vi "Initialize.vi"(8 "error in (no error)":errorcluster, 11 "State in":T1={"State"=enum."Idle", "Start Time"=timestamp(0 s since 1904-01-01), "Configuration"={"Cycle Period"=0.0, "Ismatech"={"VISA resource name"="", "Simulated?"=FALSE, "Pump Number"=1.0, "Reverse?"=FALSE}, "Masterflex"={"VISA resource name"="", "Simulated?"=FALSE, "Pump Number"=1.0, "Reverse?"=FALSE}, "Mettler"={"VISA resource name"="", "Simulated?"=FALSE}, "Bronkhorst M13 Flow Meter"={"VISA resource name"="", "Simulated?"=FALSE}, "PID 2 Parameters"={"Input Device"=enum."Bronkhorst M13", "Output Device"=enum."Ismatec ISM 831C", "Setpoint"=0.0, "PID gains"={"proportional gain (Kc)"=1.0, "integral time (Ti, min)"=0.01, "derivative time (Td, min)"=0.0}}, "Manual Entry"=0.0, "Auto?"=TRUE, "output range"={"output high"=100.0, "output low"=0.0}, "Bronkhorst M14"={"VISA resource name"="", "Simulated?"=FALSE}, "Tacmina Settings"={"Analog DAQ Task"="", "Digital DAQ Task"=""}, "KNF SIMDOS Settings"={"VISA resource name"="", "Simulated?"=TRUE}, "ASIA Pump C"={"ASIA Pump #"=0, "channel"=0, "Simulated"=FALSE}, "VICI Settings"={"VISA resource name"="", "Simulated?"=FALSE, "Pump Letter"="", "Reverse?"=FALSE}, "FLOM Settings"={"VISA resource name"="", "Simulated?"=TRUE, "Pump Number"=0.0}, "SSI PR Settings"={"VISA resource name"="", "Simulated?"=FALSE}}, "Current Time"=timestamp(0 s since 1904-01-01), "PID 1 Parameters"={"Setpoint"=0.0, "PID gains"={"proportional gain (Kc)"=1.0, "integral time (Ti, min)"=0.01, "derivative time (Td, min)"=0.0}}, "First Iteration"=FALSE, "Data"={"Flowmeter Output"=0.0, "Density"=0.0, "FL Temp"=0.0, "Scale Output (g)"=0.0, "Scale Rate of Change (g/min)"=0.0, "PID 1 Output"=0.0, "PID 2 Process Variable"=0.0, "PID 2 output"=0.0, "Pump Flow"=0.0, "Pump Pressure"=0.0}, "Process Name"="", "Pump On?"=enum."Off", "Input Error"=FALSE, "Output Error"=FALSE, "Log Started"=FALSE, "Current Setpoint"=0.0} {"PID 1 Parameters"."PID gains"."derivative time (Td, min)" format="%.3f"; "PID 1 Parameters"."PID gains"."integral time (Ti, min)" format="%.3f"; "PID 1 Parameters"."PID gains"."proportional gain (Kc)" format="%.3f"; "Configuration"."output range"."output low" min=0.0 max=100.0 format="%.2f"; "Configuration"."output range"."output high" format="%.2f"; "Configuration"."PID 2 Parameters"."PID gains"."derivative time (Td, min)" format="%.3f"; "Configuration"."PID 2 Parameters"."PID gains"."integral time (Ti, min)" format="%.3f"; "Configuration"."PID 2 Parameters"."PID gains"."proportional gain (Kc)" format="%.3f"; "Configuration"."ASIA Pump C"."channel" min=0 max=1 step=1; "Configuration"."Ismatech"."Pump Number" min=1.0 max=20.0 step=1.0; "Configuration"."Masterflex"."Pump Number" min=1.0 max=20.0 step=1.0}) -> (0 "error out":errorcluster, 1 "Pump Initialized":bool, 3 "State out":T1={"State"=enum."Idle", "Start Time"=timestamp(0 s since 1904-01-01), "Configuration"={"Cycle Period"=0.0, "Ismatech"={"VISA resource name"="", "Simulated?"=FALSE, "Pump Number"=1.0, "Reverse?"=FALSE}, "Masterflex"={"VISA resource name"="", "Simulated?"=FALSE, "Pump Number"=1.0, "Reverse?"=FALSE}, "Mettler"={"VISA resource name"="", "Simulated?"=FALSE}, "Bronkhorst M13 Flow Meter"={"VISA resource name"="", "Simulated?"=FALSE}, "PID 2 Parameters"={"Input Device"=enum."Bronkhorst M13", "Output Device"=enum."Ismatec ISM 831C", "Setpoint"=0.0, "PID gains"={"proportional gain (Kc)"=1.0, "integral time (Ti, min)"=0.01, "derivative time (Td, min)"=0.0}}, "Manual Entry"=0.0, "Auto?"=TRUE, "output range"={"output high"=100.0, "output low"=0.0}, "Bronkhorst M14"={"VISA resource name"="", "Simulated?"=FALSE}, "Tacmina Settings"={"Analog DAQ Task"="", "Digital DAQ Task"=""}, "KNF SIMDOS Settings"={"VISA resource name"="", "Simulated?"=TRUE}, "ASIA Pump C"={"ASIA Pump #"=0, "channel"=0, "Simulated"=FALSE}, "VICI Settings"={"VISA resource name"="", "Simulated?"=FALSE, "Pump Letter"="", "Reverse?"=FALSE}, "FLOM Settings"={"VISA resource name"="", "Simulated?"=TRUE, "Pump Number"=0.0}, "SSI PR Settings"={"VISA resource name"="", "Simulated?"=FALSE}}, "Current Time"=timestamp(0 s since 1904-01-01), "PID 1 Parameters"={"Setpoint"=0.0, "PID gains"={"proportional gain (Kc)"=1.0, "integral time (Ti, min)"=0.01, "derivative time (Td, min)"=0.0}}, "First Iteration"=FALSE, "Data"={"Flowmeter Output"=0.0, "Density"=0.0, "FL Temp"=0.0, "Scale Output (g)"=0.0, "Scale Rate of Change (g/min)"=0.0, "PID 1 Output"=0.0, "PID 2 Process Variable"=0.0, "PID 2 output"=0.0, "Pump Flow"=0.0, "Pump Pressure"=0.0}, "Process Name"="", "Pump On?"=enum."Off", "Input Error"=FALSE, "Output Error"=FALSE, "Log Started"=FALSE, "Current Setpoint"=0.0} {"PID 1 Parameters"."PID gains"."derivative time (Td, min)" format="%.3f"; "PID 1 Parameters"."PID gains"."integral time (Ti, min)" format="%.3f"; "PID 1 Parameters"."PID gains"."proportional gain (Kc)" format="%.3f"; "Configuration"."output range"."output low" min=0.0 max=100.0 format="%.2f"; "Configuration"."output range"."output high" format="%.2f"; "Configuration"."PID 2 Parameters"."PID gains"."derivative time (Td, min)" format="%.3f"; "Configuration"."PID 2 Parameters"."PID gains"."integral time (Ti, min)" format="%.3f"; "Configuration"."PID 2 Parameters"."PID gains"."proportional gain (Kc)" format="%.3f"; "Configuration"."ASIA Pump C"."channel" min=0 max=1 step=1; "Configuration"."Ismatech"."Pump Number" min=1.0 max=20.0 step=1.0; "Configuration"."Masterflex"."Pump Number" min=1.0 max=20.0 step=1.0})   [LabVIEW 2018, in "Feed Module.lvlib" / "Feed Module Engine.lvlib"]
uses:
  Feed Module Engine.lvlib
  State Cluster.ctl
  State Enum.ctl
  Feed Module/Controls/Feed Module Settings Cluster.ctl
  Ismatec ISM 831C/Controls/Ismatech Settings Cluster.ctl
  Masterflex 7550-30/Controls/Settings Cluster.ctl
  Mettler Toledo/Controls/Settings Cluster.ctl
  Bronkhorst M13 Flow Meter/Settings Cluster.ctl
  PID 2 Parameters Cluster.ctl
  PID Input Enum.ctl
  PID 2 Output Enum.ctl
  Tacmina QI/Tacmina QI DAQ Setting.ctl
  KNF Pump/Settings Cluster plus SIMDOS.ctl
  ASIA Pump/Pump Settings.ctl
  VICI M50 Party Mode/Settings Cluster.ctl
  FLOM Pump/Settings Cluster.ctl
  SSI PR Class/SSI PR Settings Cluster.ctl
  PID 1 Parameters Cluster.ctl
  Pump Module Folder/Measure Instrument/Pump Settings Cluster.ctl
  Tag VIs/Tag FGV Operation Enum.ctl
  Mettler Toledo/Mettler Toledo.lvlib
  Bronkhorst M13 Flow Meter/Bronkhorst M13 Flow Meter.lvlib
  Shared Variables/Dynamic Shared Variables.lvlib
  Bronkhorst M14 Flow Meter/Bronkhorst M14 Flow Meter.lvlib
  Pump Module Folder/Measure Instrument/Pump Module Engine.lvlib
  SSI PR Class/SSI PR Pump.lvlib
  FLOM Pump/FLOM Pump.lvlib
  ASIA Pump.lvlib
  KNF Pump/KNF SIMDOS.lvlib
  Tacmina QI/Tacmina QI.lvlib
  VICI M50 Party Mode/VICI M6 M50 Party Mode.lvlib
  Ismatec ISM 831C/Ismatec ISM 831C.lvlib
  Masterflex 7550-30/Masterflex 7550-30.lvlib
  Pump Module Folder/Pump Module.lvlib
  Feed Module/Feed Module.lvlib
panel:
  out "Input Initialized":bool
  # "Output Instruments"
  # "Input Instruments"
  # "Output Instruments"
  # "Input Instruments"
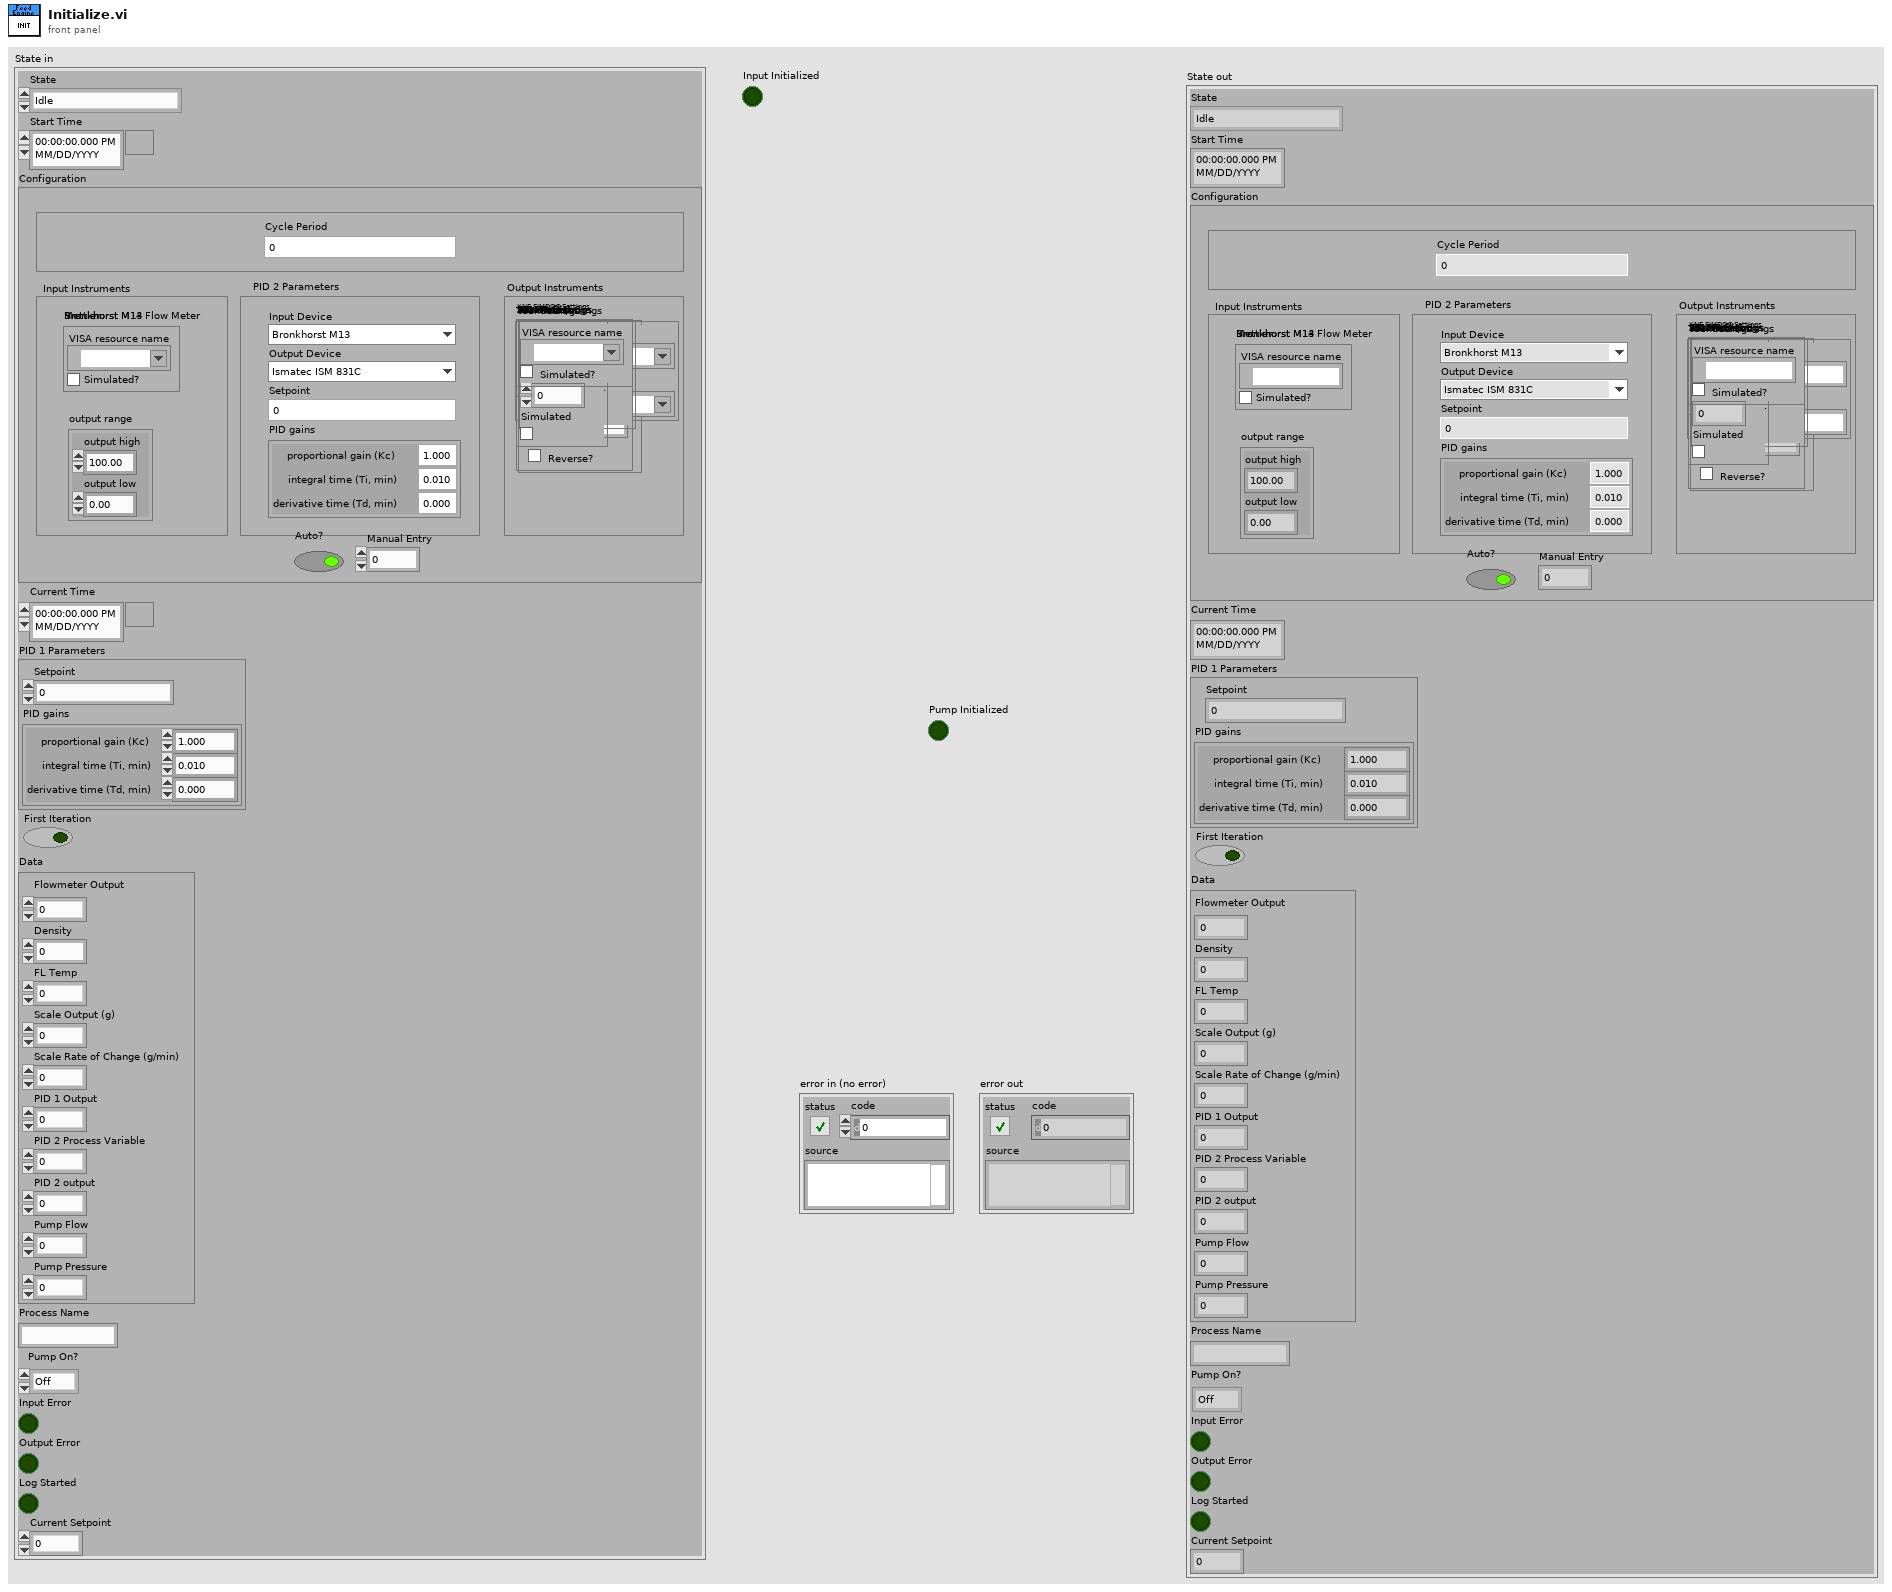
[diagram p1: front panel]
types:
  T1 = typedef "Feed Module.lvlib/Feed Module Engine.lvlib/State Cluster.ctl" = cluster{"State":T2, "Start Time":timestamp, "Configuration":T3, "Current Time":timestamp, "PID 1 Parameters":T17, "First Iteration":bool, "Data":cluster{"Flowmeter Output":dbl, "Density":dbl, "FL Temp":dbl, "Scale Output (g)":dbl, "Scale Rate of Change (g/min)":dbl, "PID 1 Output":dbl, "PID 2 Process Variable":dbl, "PID 2 output":dbl, "Pump Flow":dbl, "Pump Pressure":dbl}, "Process Name":string, "Pump On?":enum16{"Off", "On", "Not Initialized"}, "Input Error":bool, "Output Error":bool, "Log Started":bool, "Current Setpoint":dbl}
  T2 = typedef "Feed Module.lvlib/Feed Module Engine.lvlib/State Enum.ctl" = enum16{"Measuring", "Idle", "Paused"}
  T3 = typedef "Feed Module.lvlib/Feed Module Settings Cluster.ctl" = cluster{"Cycle Period":dbl, "Ismatech":T4, "Masterflex":T5, "Mettler":T6, "Bronkhorst M13 Flow Meter":T7, "PID 2 Parameters":T8, "Manual Entry":dbl, "Auto?":bool, "output range":cluster{"output high":dbl, "output low":dbl}, "Bronkhorst M14":T6, "Tacmina Settings":T11, "KNF SIMDOS Settings":T12, "ASIA Pump C":T13, "VICI Settings":T14, "FLOM Settings":T15, "SSI PR Settings":T16}
  T4 = typedef "Ismatec ISM 831C.lvlib/Ismatech Settings Cluster.ctl" = cluster{"VISA resource name":refnum<visa-resource-name>, "Simulated?":bool, "Pump Number":dbl, "Reverse?":bool}
  T5 = typedef "Masterflex 7550-30.lvlib/Settings Cluster.ctl" = cluster{"VISA resource name":refnum<visa-resource-name>, "Simulated?":bool, "Pump Number":dbl, "Reverse?":bool}
  T6 = typedef "Mettler Toledo.lvlib/Settings Cluster.ctl" = cluster{"VISA resource name":refnum<visa-resource-name>, "Simulated?":bool}
  T7 = typedef "Bronkhorst M13 Flow Meter.lvlib/Settings Cluster.ctl" = cluster{"VISA resource name":refnum<visa-resource-name>, "Simulated?":bool}
  T8 = typedef "PID 2 Parameters Cluster.ctl" = cluster{"Input Device":T9, "Output Device":T10, "Setpoint":dbl, "PID gains":cluster{"proportional gain (Kc)":dbl, "integral time (Ti, min)":dbl, "derivative time (Td, min)":dbl}}
  T9 = typedef "PID Input Enum.ctl" = enum16{"Default", "Bronkhorst M13", "Bronkhorst M14", "Scale Rate of Change"}
  T10 = typedef "PID 2 Output Enum.ctl" = enum16{"Default", "Ismatec ISM 831C", "Masterflex 7550-30", "VICI", "Tacmina QI", "KNF SIMDOS", "ASIA Type C", "FLOM UI-22-11", "SSI PR"}
  T11 = typedef "Tacmina QI.lvlib/Tacmina QI DAQ Setting.ctl" = cluster{"Analog DAQ Task":refnum<k21>, "Digital DAQ Task":refnum<k21>}
  T12 = typedef "KNF SIMDOS.lvlib/Settings Cluster plus SIMDOS.ctl" = cluster{"VISA resource name":refnum<visa-resource-name>, "Simulated?":bool}
  T13 = typedef "ASIA Pump.lvlib/Pump Settings.ctl" = cluster{"ASIA Pump #":i32, "channel":i32, "Simulated":bool}
  T14 = typedef "VICI M6 M50 Party Mode.lvlib/Settings Cluster.ctl" = cluster{"VISA resource name":refnum<visa-resource-name>, "Simulated?":bool, "Pump Letter":string, "Reverse?":bool}
  T15 = typedef "FLOM Pump.lvlib/Settings Cluster.ctl" = cluster{"VISA resource name":refnum<visa-resource-name>, "Simulated?":bool, "Pump Number":dbl}
  T16 = typedef "SSI PR Pump.lvlib/SSI PR Settings Cluster.ctl" = cluster{"VISA resource name":refnum<visa-resource-name>, "Simulated?":bool}
  T17 = typedef "PID 1 Parameters Cluster.ctl" = cluster{"Setpoint":dbl, "PID gains":cluster{"proportional gain (Kc)":dbl, "integral time (Ti, min)":dbl, "derivative time (Td, min)":dbl}}
  T18 = typedef "Pump Module.lvlib/Pump Settings Cluster.ctl" = cluster{"Output Device":T10, "Masterflex":T5, "Ismatech":T4, "VICI Settings":T14, "Tacmina Settings":T11, "KNF SIMDOS Settings":T12, "ASIA Pump C":T13, "FLOM Settings":T15, "SSI PR Settings":T16}
  T19 = typedef "Tag FGV Operation Enum.ctl" = enum16{"Init", "Set Notification Queue", "Create Tag", "Commit", "Write Tag (Numeric)", "Write Tag (Boolean)", "Read All Tags", "Read One Tag", "Delete Tag Category", "Set Alarm Parameters (Numeric)", "Set Alarm Parameters (Boolean)", "Enable All Alarms", "Disable All Alarms", "Delete All Tags", "Read Alarms", "Ack Alarm", "Read Alarm Parameters (Numeric)", "Read Alarm Parameters (Boolean)"}
  T20 = typedef "Feed Module.lvlib/Feed Module Tag Names Cluster.ctl" = cluster{"Pump Flow Tag":string, "PID 2 Out Tag":string, "Scale Tag":string, "Density Tag":string, "FL Temp":string, "Input Device Tag":string, "Output Device Tag":string, "Pump's Flow":string, "Pump's Pressure":string, "Overpressure Tag":string}
  T21 = typedef "Bronkhorst M14 Flow Meter.lvlib/Settings Cluster.ctl" = cluster{"VISA resource name":refnum<visa-resource-name>, "Simulated?":bool}
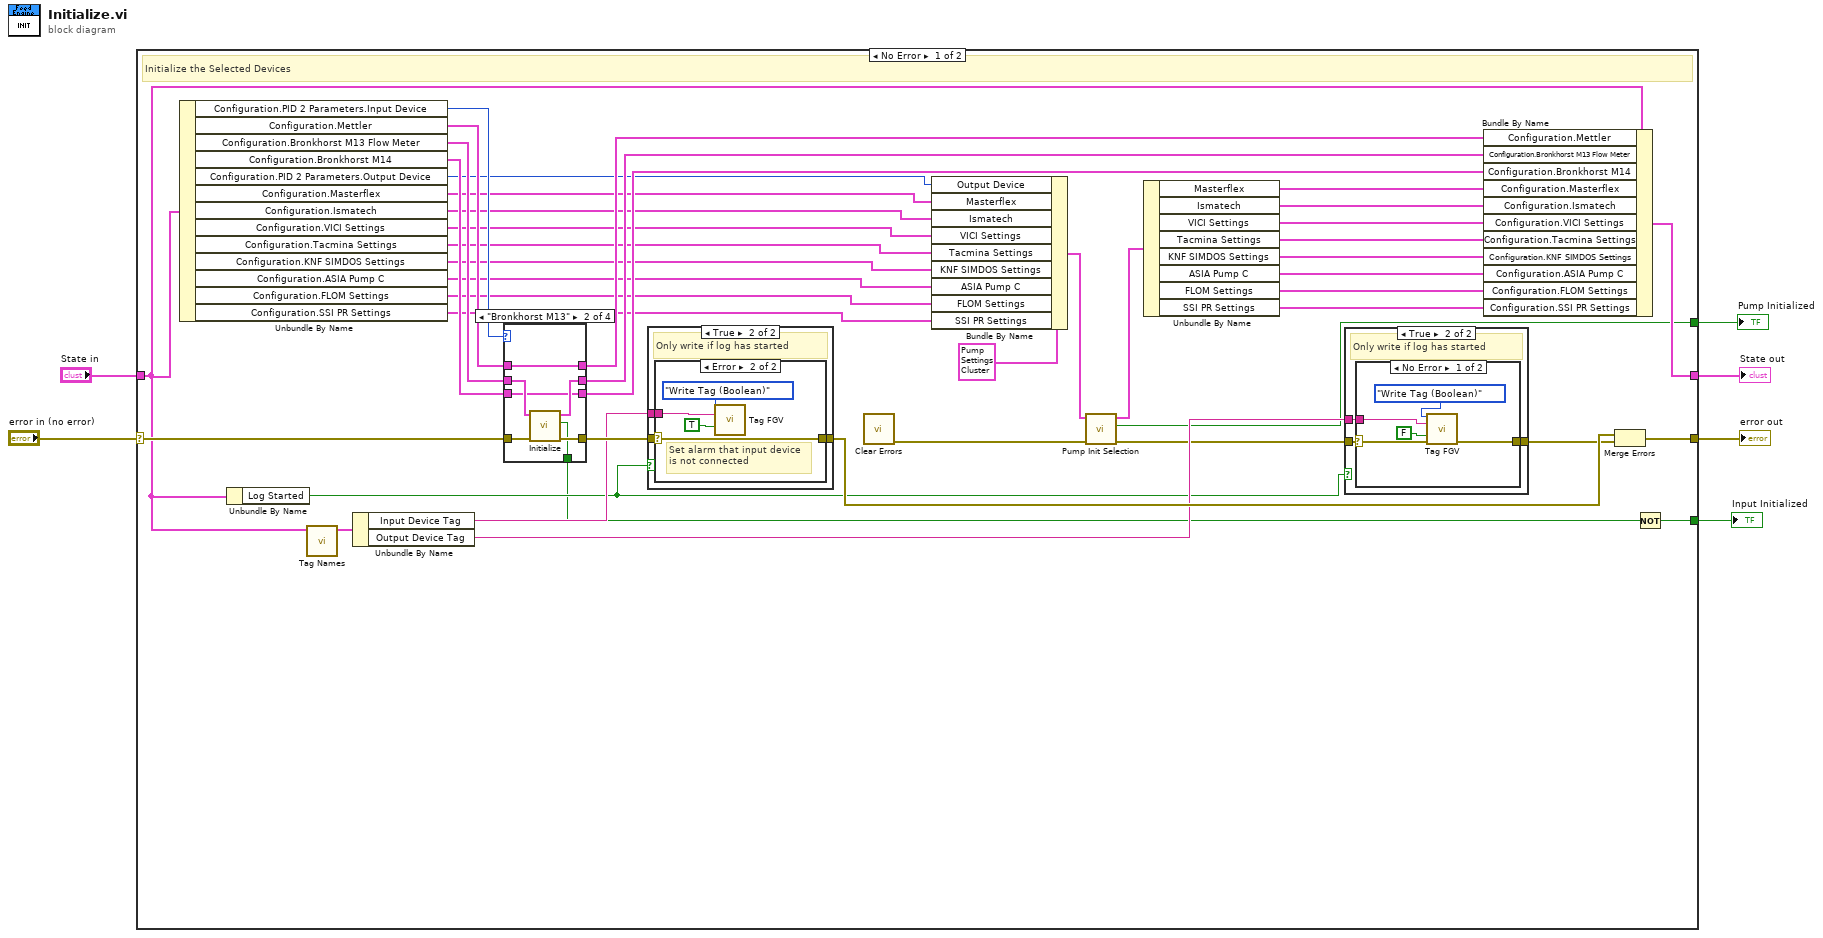
[diagram p0: block diagram]
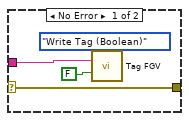
[diagram p3: hidden frame]
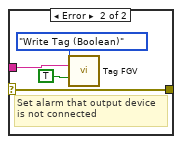
[diagram p5: hidden frame]
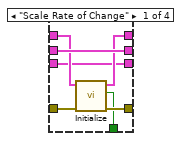
[diagram p6: hidden frame]
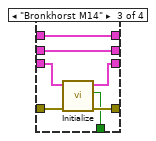
[diagram p7: hidden frame]
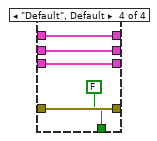
[diagram p8: hidden frame]
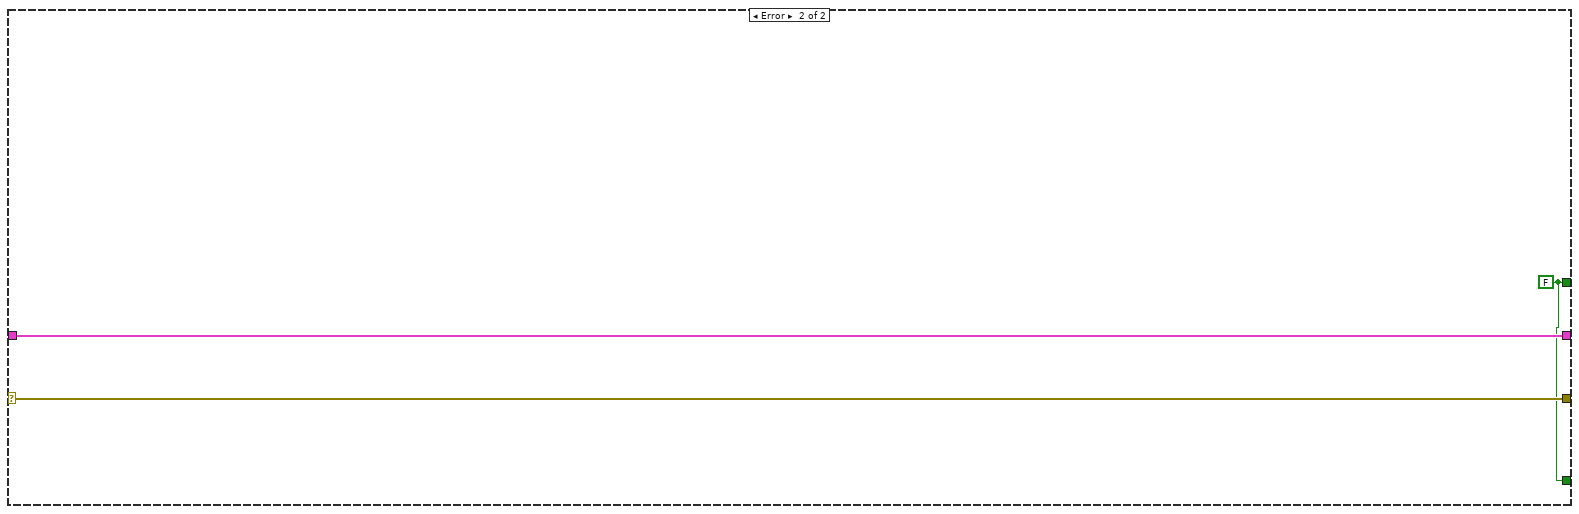
[diagram p9: hidden frame]
diagram:
  n1 = case shown="No Error" "error in (no error)" {
    selector: "error in (no error)" -> [w46 w103]
    tunnel: [w38 w103] -> w5
    tunnel: "State in" -> [w32 w102]
    tunnel: [w44 w102] -> w3
    tunnel: [w11 w101] -> w2
    tunnel: [w7 w101] -> w1
    frame No Error {
      # "Initialize the Selected Devices"
      n2 = Unbundle By Name(w32) -> ("Configuration.PID 2 Parameters.Input Device"=w49:T9, "Configuration.Mettler"=w48:T6, "Configuration.Bronkhorst M13 Flow Meter"=w47:T7, "Configuration.Bronkhorst M14"=w34:T6, "Configuration.PID 2 Parameters.Output Device"=w30:T10, "Configuration.Masterflex"=w27:T5, "Configuration.Ismatech"=w26:T4, "Configuration.VICI Settings"=w25:T14, "Configuration.Tacmina Settings"=w24:T11, "Configuration.KNF SIMDOS Settings"=w23:T12, "Configuration.ASIA Pump C"=w22:T13, "Configuration.FLOM Settings"=w21:T15, "Configuration.SSI PR Settings"=w20:T16)
      n3 = Unbundle By Name(w32) -> ("Log Started"=w33:bool)
      n4 = call "Tag Names.vi"("State in"=w32) -> ("Feed Module Tag Names"=w41:T20)  [unwired: 6 in, 4 out]
      n5 = Unbundle By Name(w41) -> ("Input Device Tag"=w40:string, "Output Device Tag"=w36:string)
      n6 = case shown="\"Bronkhorst M13\"" w49 {
        tunnel: w48 -> [w78 w88 w95 w100]
        tunnel: w47 -> [w81 w87 w92 w99]
        tunnel: w46 -> [w77 w86 w94 w98]
        tunnel: [w79 w85 w93 w98] -> w42
        tunnel: [w81 w84 w92 w99] -> w45
        tunnel: [w80 w88 w95 w100] -> w43
        tunnel: w34 -> [w76 w83 w91 w97]
        tunnel: [w76 w83 w90 w97] -> w35
        tunnel: [w75 w82 w89 FALSE ("No Meter Connected")] -> w8
        frame "Scale Rate of Change" {
          n7 = call "Initialize.vi"("error in (no error)"=w77, "Mettler Settings in"=w78) -> ("error out"=w79:errorcluster, "No Scale Connected"=w75:bool, "Mettler Settings out"=w80:T6)  [unwired: 7 in]
        }
        frame "Bronkhorst M13" {
          n8 = call "Initialize.vi"("error in (no error)"=w86, "Bronkhorst Settings in"=w87) -> ("error out"=w85:errorcluster, "No Meter Connnected"=w82:bool, "Bronkhorst Settings out"=w84:T7)  [unwired: 7 in]
        }
        frame "Bronkhorst M14" {
          n9 = call "Initialize.vi"("error in (no error)"=w94, "Bronkhorst Settings in"=w91) -> ("error out"=w93:errorcluster, "No Meter Connected"=w89:bool, "Bronkhorst Settings out"=w90:T21)  [unwired: 7 in]
        }
        frame "Default", Default {
        }
      }
      n10 = case shown="True" w33 {
        tunnel: w42 -> [w50 w53]
        tunnel: w40 -> [_ w52]
        tunnel: [w50 w51] -> w39
        frame False {
        }
        frame True {
          # "Only write if log has started"
          n11 = case shown="Error" w53 {
            selector: w53 -> [w54 w59]
            tunnel: [w54 w59] -> w51
            tunnel: w52 -> [w55 w58]
            frame No Error {
              n12 = call "Tag FGV.vi"("Operation"=Tag_FGV_Operation_Enum."Write Tag (Boolean)", "Tag Name"=w55, "Data"=FALSE) -> ()  [unwired: 5 in, 8 out]
            }
            frame Error {
              # "Set alarm that input device\nis not connected"
              n13 = call "Tag FGV.vi"("Operation"=Tag_FGV_Operation_Enum."Write Tag (Boolean)", "Tag Name"=w58, "Data"=TRUE) -> ()  [unwired: 5 in, 8 out]
            }
          }
        }
      }
      n14 = call <vilib>:"Clear Errors.vi"() -> ("error out"=w31:errorcluster)  [unwired: 6 in, 1 out]
      n15 = Bundle By Name(cluster=T18 {"Output Device"=enum."Default", "Masterflex"={"VISA resource name"="", "Simulated?"=FALSE, "Pump Number"=0.0, "Reverse?"=FALSE}, "Ismatech"={"VISA resource name"="", "Simulated?"=FALSE, "Pump Number"=0.0, "Reverse?"=FALSE}, "VICI Settings"={"VISA resource name"="", "Simulated?"=FALSE, "Pump Letter"="", "Reverse?"=FALSE}, "Tacmina Settings"={"Analog DAQ Task"="", "Digital DAQ Task"=""}, "KNF SIMDOS Settings"={"VISA resource name"="", "Simulated?"=FALSE}, "ASIA Pump C"={"ASIA Pump #"=0, "channel"=0, "Simulated"=FALSE}, "FLOM Settings"={"VISA resource name"="", "Simulated?"=FALSE, "Pump Number"=0.0}, "SSI PR Settings"={"VISA resource name"="", "Simulated?"=FALSE}}, "Output Device"=w30, "Masterflex"=w27, "Ismatech"=w26, "VICI Settings"=w25, "Tacmina Settings"=w24, "KNF SIMDOS Settings"=w23, "ASIA Pump C"=w22, "FLOM Settings"=w21, "SSI PR Settings"=w20) -> (w29:T18)
      n16 = call "Pump Init Selection.vi"("error in (no error)"=w31, "Pump Settings In"=w29) -> ("error out"=w10:errorcluster, "Initialized"=w11:bool, "Pump Settings Out"=w28:T18)  [unwired: 7 in]
      n17 = Unbundle By Name(w28) -> ("Masterflex"=w19:T5, "Ismatech"=w18:T4, "VICI Settings"=w17:T14, "Tacmina Settings"=w16:T11, "KNF SIMDOS Settings"=w15:T12, "ASIA Pump C"=w14:T13, "FLOM Settings"=w13:T15, "SSI PR Settings"=w12:T16)
      n18 = case shown="True" w33 {
        tunnel: w10 -> [w62 w65]
        tunnel: [w62 w64] -> w37
        tunnel: w36 -> [_ w63]
        frame False {
        }
        frame True {
          # "Only write if log has started"
          n19 = case shown="No Error" w65 {
            selector: w65 -> [w67 w72]
            tunnel: [w66 w72] -> w64
            tunnel: w63 -> [w68 w71]
            frame No Error {
              n20 = call "Tag FGV.vi"("Operation"=Tag_FGV_Operation_Enum."Write Tag (Boolean)", "Tag Name"=w68, "Data"=FALSE, "error in (no error)"=w67) -> ("error out"=w66:errorcluster)  [unwired: 4 in, 7 out]
            }
            frame Error {
              # "Set alarm that output device\nis not connected"
              n21 = call "Tag FGV.vi"("Operation"=Tag_FGV_Operation_Enum."Write Tag (Boolean)", "Tag Name"=w71, "Data"=TRUE) -> ()  [unwired: 5 in, 8 out]
            }
          }
        }
      }
      n22 = Bundle By Name(cluster=w32, "Configuration.Mettler"=w43, "Configuration.Bronkhorst M13 Flow Meter"=w45, "Configuration.Bronkhorst M14"=w35, "Configuration.Masterflex"=w19, "Configuration.Ismatech"=w18, "Configuration.VICI Settings"=w17, "Configuration.Tacmina Settings"=w16, "Configuration.KNF SIMDOS Settings"=w15, "Configuration.ASIA Pump C"=w14, "Configuration.FLOM Settings"=w13, "Configuration.SSI PR Settings"=w12) -> (w44:T1)
      n23 = Merge Errors(w39, w37) -> (w38:errorcluster)
      n24 = Not(x=w8) -> (.not. x?=w7:bool)
    }
    frame Error {
      w101 = FALSE ("Initialized")
    }
  }
  "error out" <- w5
  "State out" <- w3
  "Pump Initialized" <- w2
  "Input Initialized" <- w1
